vi "02_moreBasics.vi"() -> ()   [LabVIEW 2011]
panel:
  in  "ArrayIn":i32[](array[numeric])=[1, 4, 0]
  out "current state":enum16{"init", "run", "error", "stop"}(ring)
  in  "running":bool
  # "change 02_array.vi, s.t. any non-zero is an error\nchange vi's that they accept 2d arrays\nAdd error dialog if error (and see why not to use them)\nAdd matrix indices to error string"
  # "off"
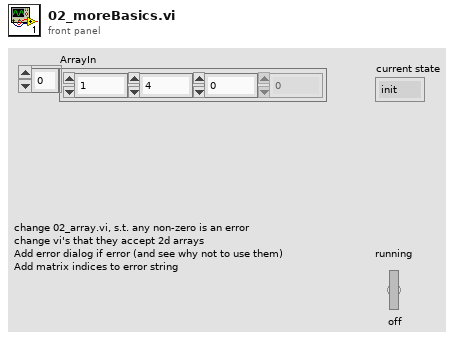
[diagram p1: front panel]
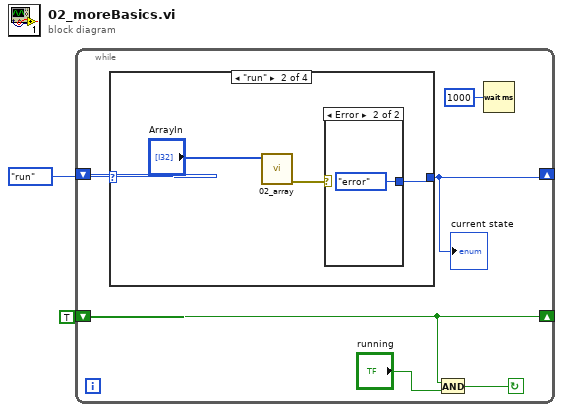
[diagram p0: block diagram]
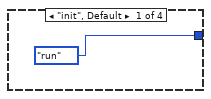
[diagram p2: hidden frame]
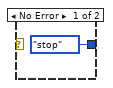
[diagram p3: hidden frame]
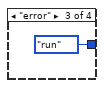
[diagram p4: hidden frame]
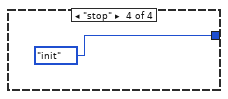
[diagram p5: hidden frame]
diagram:
  n1 = while {
    shift-right: [w6] -> _
    shift-left: TRUE -> [w6]
    shift-right: [w4] -> _
    shift-left: enum16{"init", "run", "error", "stop"}."run" ("state") -> [w5]
    stop <- w7 continue-if-true
    n2 = case shown="\"run\"" w5 {
      tunnel: [enum16{"init", "run", "error", "stop"}."run" ("state") w12 enum16{"init", "run", "error", "stop"}."run" ("state") enum16{"init", "run", "error", "stop"}."init" ("state")] -> w4
      frame "init", Default {
      }
      frame "run" {
        n3 = call "02_array.vi"("ArrayIn"="ArrayIn") -> ("errorOut"=w10:errorcluster)  [unwired: 9 in, 1 out]
        n4 = case shown="Error" w10 {
          tunnel: [enum16{"init", "run", "error", "stop"}."stop" ("state") enum16{"init", "run", "error", "stop"}."error" ("state")] -> w12
          frame No Error {
          }
          frame Error {
          }
        }
      }
      frame "error" {
      }
      frame "stop" {
      }
    }
    "current state" <- w4
    n5 = And(x=w6, y="running") -> (x .and. y?=w7:bool)
    n6 = Wait (ms)(milliseconds to wait=u32 1000) -> ()  [unwired: 1 out]
  }
